vi "plugin_call.vi"(4 "Data":variant, 5 "Path":path, 6 "Section":string, 7 "vi":string="blinker") -> (0 "error out":errorcluster)   [LabVIEW 2010]
uses:
  <vilib>/Utility/config.llb/Read Key (String).vi
  <vilib>/Utility/config.llb/NI_LVConfig.lvlib
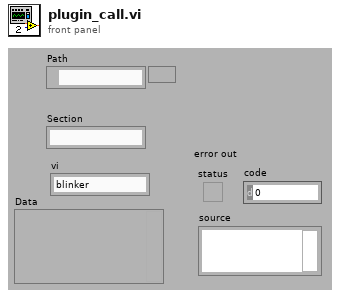
[diagram p1: front panel]
types:
  T1 = typedef "NI_LVConfig.lvlib/Config Data RefNum.ctl" = refnum<k1>
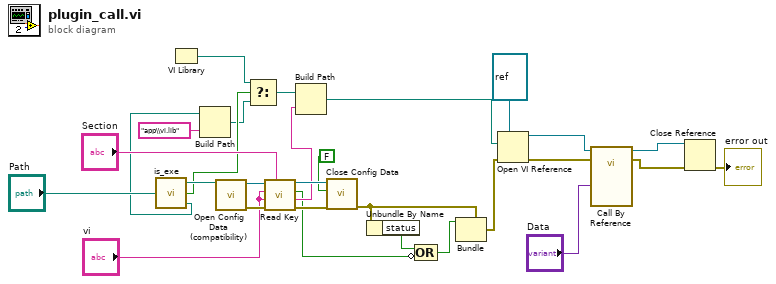
[diagram p0: block diagram]
diagram:
  n1 = call "is_exe.vi"("path"="Path") -> ("actual path"=w3:path, "exe?"=w20:bool, "ini path"=w26:path)  [unwired: 2 in]
  n2 = VI Library() -> (path=w19:path)
  n3 = Build Path(base path=w3, name or relative path="app\\vi.lib") -> (appended path=w2:path)
  n4 = call <vilib>:"Open Config Data (compatibility).vi"("configuration file path"=w26) -> ("error out"=w28:errorcluster, "refnum"=w27:T1)  [unwired: 8 in, 1 out]
  n5 = Select(t=w19, s=w20, f=w2) -> (s? t:f=w18:path)
  n6 = call-poly <vilib>:"Read Key.vi"("section"="Section", "error in (no error)"=w28, "default value"="vi", "key"="vi", "refnum"=w27) -> ("error out"=w24:errorcluster, "value"=w17:string, "found?"=w13:bool, "refnum out"=w23:T1)  [unwired: 3 in]
  n7 = Build Path(base path=w18, name or relative path=w17) -> (appended path=w11:path)
  n8 = call <vilib>:"Close Config Data.vi"("error in (no error)"=w24, "write file if changed (T)"=FALSE ("write configuration file? (T)"), "refnum"=w23) -> ("error out"=w16:errorcluster)  [unwired: 7 in, 1 out]
  n9 = Unbundle By Name(w16) -> ("status"=w15:bool)
  n10 = Compound Arithmetic op=OR(w15, invert w13) -> (w14:bool)
  n11 = Bundle(cluster=w16, "status"=w14) -> (w12:errorcluster)  [unwired: 2 in]
  n12 = Open VI Reference(type specifier VI Refnum (for type only)=refnum<vi> refnum, vi path=w11, error in (no error)=w12) -> (vi reference=w9:refnum<vi>, error out=w10:errorcluster)  [unwired: 3 in]
  n13 = call-by-ref "?"(reference=w9, error in=w10, "Variant"="Data") -> (reference out=w8:refnum<vi>, error out=w7:errorcluster)
  n14 = Close Reference(reference=w8, error in (no error)=w7) -> (error out=→"error out":errorcluster)
